vi "MTS_ShowHideTabs.vi"(7 "Action":enum16{"Show All", "Hide Tab", "Show Tab"}(ring), 8 "error in (no error)":errorcluster, 10 "Tab Caption":string, 11 "ShowTab":refnum<vi>) -> (0 "error out":errorcluster, 3 "ShowTab":refnum<vi>)   [LabVIEW 2011]
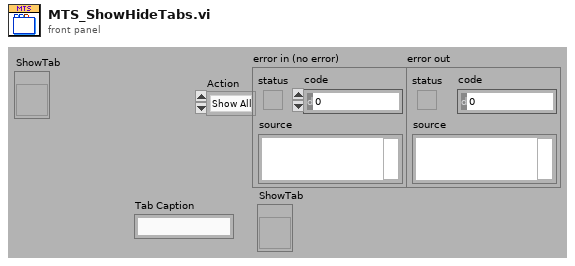
[diagram p1: front panel]
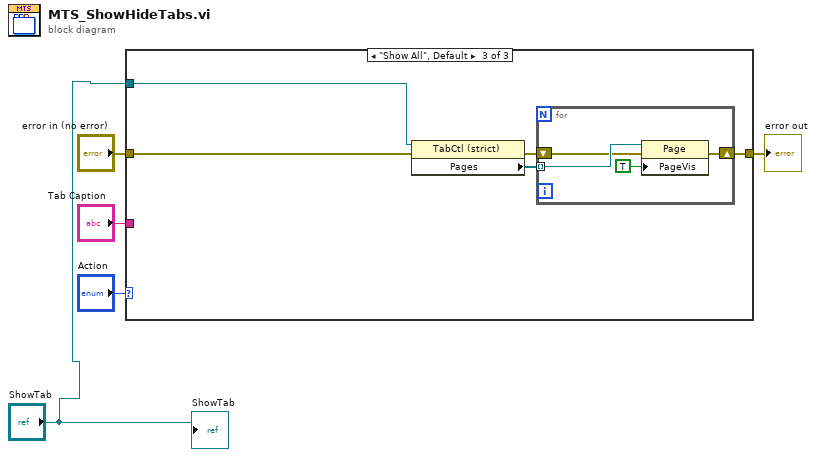
[diagram p0: block diagram]
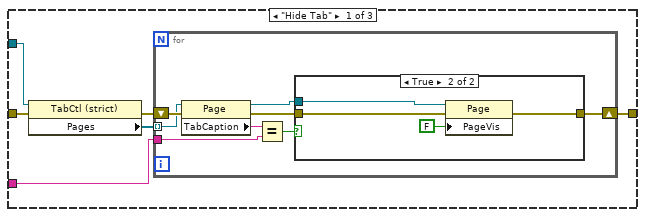
[diagram p2: hidden frame]
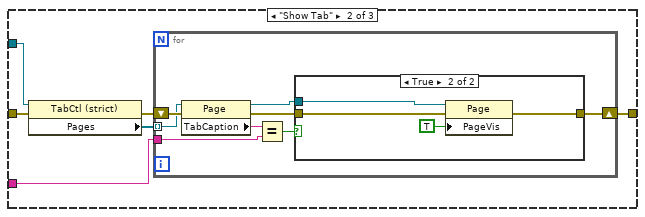
[diagram p4: hidden frame]
diagram:
  n1 = case shown="\"Show All\", Default" "Action" {
    tunnel: "ShowTab" -> [w11 w30 w48]
    tunnel: "error in (no error)" -> [w8 w27 w45]
    tunnel: [w7 w26 w44] -> w4
    tunnel: "Tab Caption" -> [w6 w25 _]
    frame "Hide Tab" {
      n2 = property on="Property Node" class="TabCtl (strict)"(reference=w11, error in=w8) -> (error out=w9:errorcluster, "Pages"=w10:refnum<vi>[])  [unwired: 1 out]
      n3 = for {
        tunnel: w10 -> [w18] mode=indexing
        shift-right: [w13] -> w7
        shift-left: w9 -> [w19]
        tunnel: w6 -> [w16]
        n4 = property on="Property Node" class="Page"(reference=w18, error in=w19) -> (reference out=w14:refnum<vi>, error out=w15:errorcluster, "TabCaption"=w17:string)
        n5 = Equal?(x=w17, y=w16) -> (x = y?=w12:bool)
        n6 = case shown="True" w12 {
          tunnel: w15 -> [w20 w24]
          tunnel: w14 -> [_ w23]
          tunnel: [w20 w22] -> w13
          frame False {
          }
          frame True {
            n7 = property on="Property Node" class="Page"(reference=w23, error in=w24, "PageVis"=FALSE ("Page Visible")) -> (error out=w22:errorcluster)  [unwired: 1 out]
          }
        }
      }
    }
    frame "Show Tab" {
      n8 = property on="Property Node" class="TabCtl (strict)"(reference=w30, error in=w27) -> (error out=w28:errorcluster, "Pages"=w29:refnum<vi>[])  [unwired: 1 out]
      n9 = for {
        tunnel: w29 -> [w37] mode=indexing
        shift-right: [w32] -> w26
        shift-left: w28 -> [w38]
        tunnel: w25 -> [w35]
        n10 = property on="Property Node" class="Page"(reference=w37, error in=w38) -> (reference out=w33:refnum<vi>, error out=w34:errorcluster, "TabCaption"=w36:string)
        n11 = Equal?(x=w36, y=w35) -> (x = y?=w31:bool)
        n12 = case shown="True" w31 {
          tunnel: w34 -> [w39 w43]
          tunnel: w33 -> [_ w42]
          tunnel: [w39 w41] -> w32
          frame False {
          }
          frame True {
            n13 = property on="Property Node" class="Page"(reference=w42, error in=w43, "PageVis"=TRUE ("Page Visible")) -> (error out=w41:errorcluster)  [unwired: 1 out]
          }
        }
      }
    }
    frame "Show All", Default {
      n14 = property on="Property Node" class="TabCtl (strict)"(reference=w48, error in=w45) -> (error out=w46:errorcluster, "Pages"=w47:refnum<vi>[])  [unwired: 1 out]
      n15 = for {
        tunnel: w47 -> [w51] mode=indexing
        shift-right: [w52] -> w44
        shift-left: w46 -> [w50]
        n16 = property on="Property Node" class="Page"(reference=w51, error in=w50, "PageVis"=TRUE ("Page Visible")) -> (error out=w52:errorcluster)  [unwired: 1 out]
      }
    }
  }
  "error out" <- w4
  "ShowTab" <- "ShowTab"
